vi "Test - Texture Mapping Test 1.vi"() -> ()   [LabVIEW 2020, in "3D (FPGA).lvlib"]
uses:
  3D (FPGA).lvlib
  Libraries/Utility/Utility.lvlib
  Raster/Raster (FPGA).lvlib
  Vector 3D.ctl
  Triangle 3D With Colour.ctl
  Raster/Rectangle Dimensions.ctl
  Camera.ctl
panel:
  in  "x Rotation":sgl(slide) scale=-180.0..180.0
  in  "y Rotation":sgl(slide) scale=0.0..360.0
  in  "z Rotation":sgl(slide) scale=-180.0..180.0
  in  "x Transform":sgl(slide) scale=-10.0..10.0
  in  "y Transform":sgl(slide)=5.0 scale=-10.0..10.0
  in  "z Transform":sgl(slide)=-10.0 scale=-20.0..10.0
  out "2D Picture 2":picture
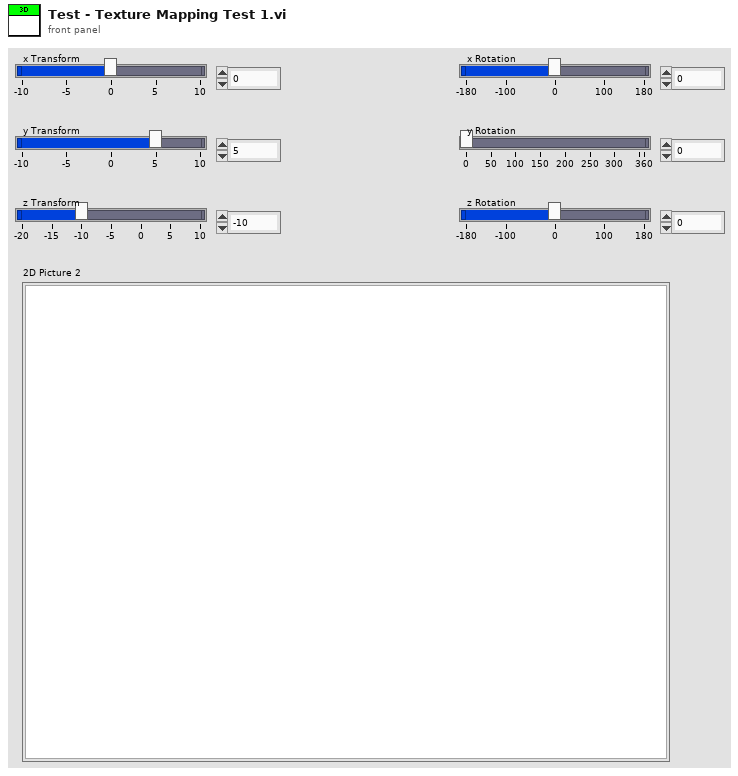
[diagram p1: front panel]
types:
  T1 = typedef "3D (FPGA).lvlib/Vector 3D.ctl" = cluster{"x":sgl, "y":sgl, "z":sgl}
  T2 = typedef "3D (FPGA).lvlib/Camera.ctl" = cluster{"Field Of View":sgl, "Near Plane":sgl, "Far Plane":sgl}
  T3 = typedef "Raster (FPGA).lvlib/Rectangle Dimensions.ctl" = cluster{"Width":u32, "Height":u32}
  T4 = typedef "3D (FPGA).lvlib/Object.ctl" = cluster{"Triangles":T5[], "Transform":T10, "Name":string, "Alpha Blending Enabled":bool, "Alpha":dbl, "Turntable Enabled":bool, "Material":T8}
  T5 = typedef "3D (FPGA).lvlib/Triangle.ctl" = cluster{"Vertex 1":T6, "Vertex 2":T6, "Vertex 3":T6, "Alpha":dbl, "Alpha Blending Enabled":bool, "Colour":u32, "Material":T8}
  T6 = typedef "3D (FPGA).lvlib/Vertex.ctl" = cluster{"Position":T1, "UV":T7, "Colour":u32}
  T7 = typedef "Raster (FPGA).lvlib/UV.ctl" = cluster{"u":sgl, "v":sgl}
  T8 = typedef "3D (FPGA).lvlib/Material.ctl" = cluster{"Diffuse Colour":u32, "Texture":T9}
  T9 = typedef "Raster (FPGA).lvlib/Texture.ctl" = cluster{"Pixels":refnum<data-value>, "Size":T3}
  T10 = typedef "3D (FPGA).lvlib/Transform.ctl" = cluster{"Position":T1, "Rotation":T1, "Scale":T1}
  T11 = typedef "3D.lvlib/Triangle 3D.ctl" = cluster{"Point 1":T12, "Point 2":T12, "Point 3":T12}
  T12 = typedef "3D.lvlib/Vector 3D.ctl" = cluster{"x":sgl, "y":sgl, "z":sgl}
  T13 = typedef "imagedata.ctl" = cluster{"image type":i32, "image depth":i32, "image":u8[], "mask":u8[], "colors":u32[], "Rectangle":cluster{"left":i16, "top":i16, "right":i16, "bottom":i16}}
  T14 = typedef "3D (FPGA).lvlib/Triangle 3D With Colour.ctl" = cluster{"Point 1":T1, "Point 2":T1, "Point 3":T1, "Fill Colour":u32, "Alpha":dbl, "Alpha Blending Enabled":bool, "Index":i32}
  T15 = typedef "3D.lvlib/Point 2D.ctl" = cluster{"x":sgl, "y":sgl}
  T16 = typedef "Raster.lvlib/UV.ctl" = cluster{"u":sgl, "v":sgl}
  T17 = typedef "Raster (FPGA).lvlib/Point 2D (I32).ctl" = cluster{"x":i32, "y":i32}
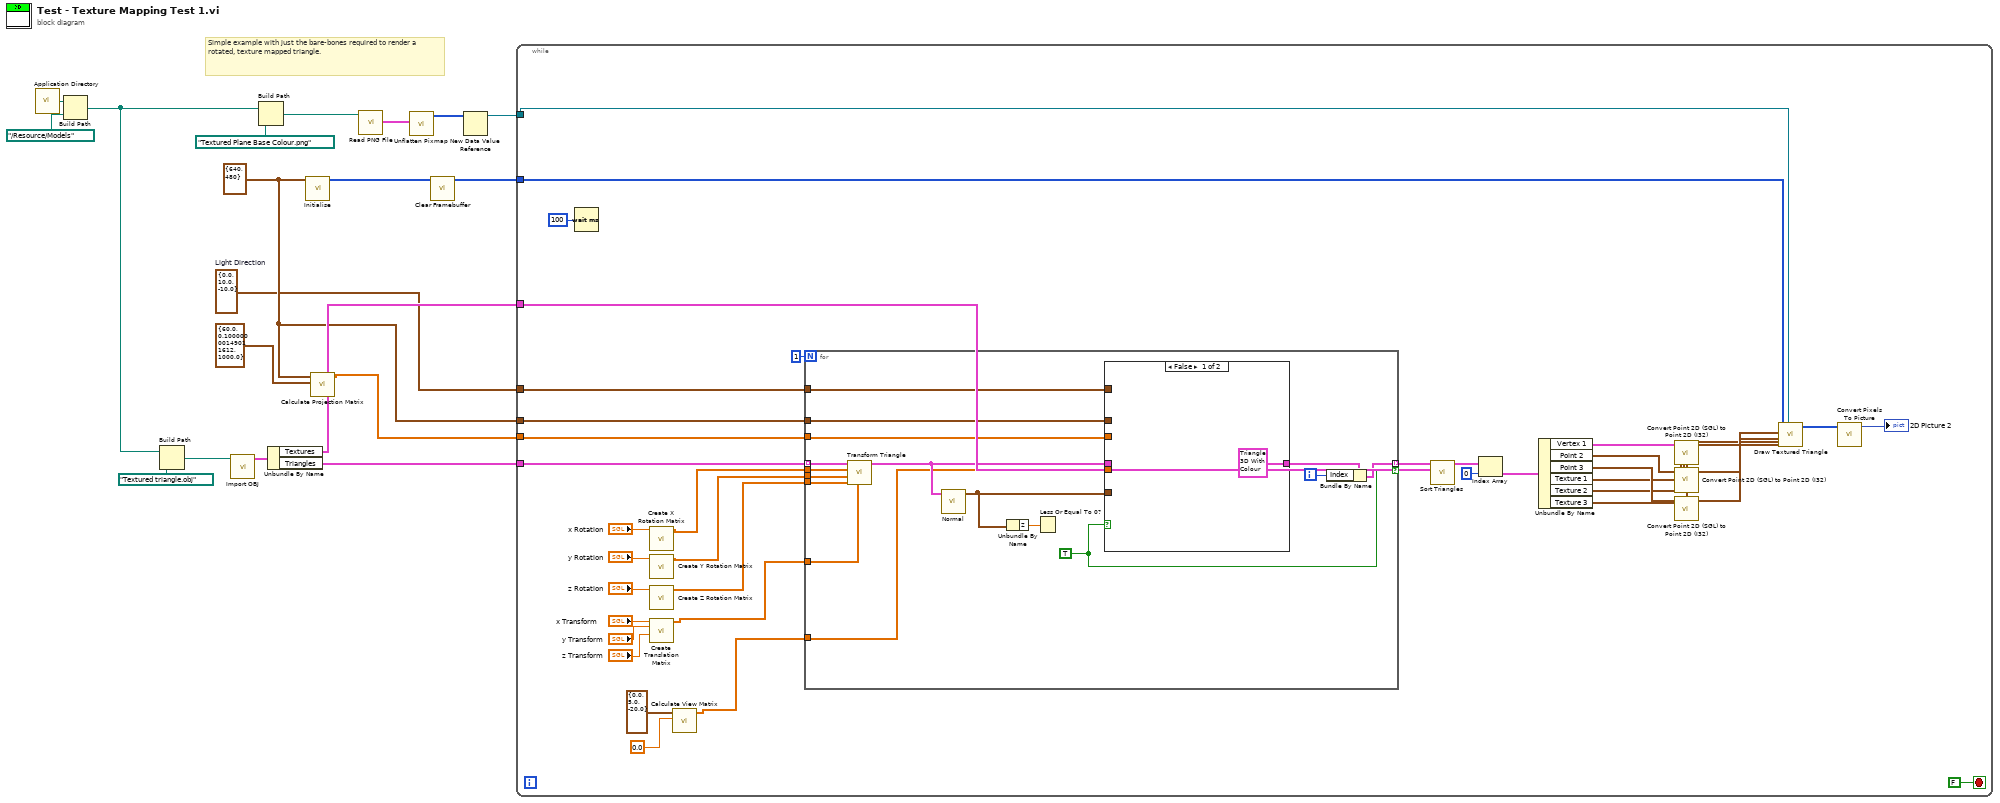
[diagram p0: block diagram]
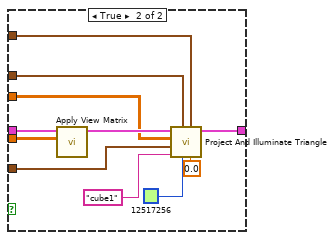
[diagram p2: hidden frame]
diagram:
  w13 = T1 {"x"=0.0, "y"=10.0, "z"=-10.0}  # Light Direction
  w14 = T3 {"Width"=640, "Height"=480} ("Screen Dimensions")
  # "Simple example with just the bare-bones required to render a rotated, texture mapped triangle."
  n1 = call <vilib>:"Application Directory.vi"() -> ("Application Directory"=w11:path)
  n2 = Build Path(base path=w11, name or relative path=path "../Resource/Models") -> (appended path=w5:path)
  n3 = Build Path(base path=w5, name or relative path=path "Textured triangle.obj") -> (appended path=w8:path)
  n4 = call "Import OBJ.vi"("Object"=w8) -> ("Object"=w18:T4)  [unwired: 9 in, 1 out]
  n5 = Build Path(base path=w5, name or relative path=path "Textured Plane Base Colour.png") -> (appended path=w6:path)
  n6 = Unbundle By Name(w18) -> ("Textures"=w15:T11[], "Triangles"=w1:T5[])
  n7 = call "Initialise.vi"("Screen Dimensions"=w14) -> ("Pixel Data out"=w16:u32[][])  [unwired: 10 in]
  n8 = call "Calculate Projection Matrix.vi"("Camera"=T2 {"Field Of View"=60.0, "Near Plane"=0.1, "Far Plane"=1000.0}, "Screen Dimensions"=w14) -> ("Projection Matrix"=w12:sgl[][])  [unwired: 9 in]
  n9 = call <vilib>:"Read PNG File.vi"("path to PNG file"=w6) -> ("image data"=w3:T13)  [unwired: 8 in, 2 out]
  n10 = call <vilib>:"Unflatten Pixmap.vi"("image data"=w3) -> ("24-bit pixmap"=w4:u32[][])  [unwired: 4 in, 6 out]
  n11 = call "Clear Framebuffer.vi"("Pixel Data in"=w16) -> ("Pixel Data out"=w19:u32[][])  [unwired: 10 in]
  n12 = New Data Value Reference(data value=w4) -> (data value reference=w2:refnum<data-value>)  [unwired: 1 in, 1 out]
  n13 = while {
    tunnel: w19 -> [w56]
    tunnel: w15 -> [w31]
    tunnel: w14 -> [w29]
    tunnel: w13 -> [w28]
    tunnel: w12 -> [w27]
    tunnel: w2 -> [w23]
    tunnel: w1 -> [w22]
    stop <- FALSE stop-if-true
    n14 = Wait (ms)(milliseconds to wait=u32 100) -> ()  [unwired: 1 out]
    n15 = call "Create X Rotation Matrix.vi"("Theta (°)"="x Rotation") -> ("Rotation X Matrix"=w39:sgl[][])  [unwired: 10 in]
    n16 = call "Create Y Rotation Matrix.vi"("Theta (°)"="y Rotation") -> ("Rotation Y Matrix"=w38:sgl[][])  [unwired: 10 in]
    n17 = call "Create Z Rotation Matrix.vi"("Theta (°)"="z Rotation") -> ("Rotation Z Matrix"=w37:sgl[][])  [unwired: 10 in]
    n18 = call "Create Translation Matrix.vi"("z"="z Transform", "y"="y Transform", "x"="x Transform") -> ("Translation Matrix"=w36:sgl[][])  [unwired: 8 in]
    n19 = call "Calculate View Matrix.vi"("Camera Rotation"=sgl 0.0, "Camera Position"=T1 {"x"=0.0, "y"=5.0, "z"=-20.0} ("output cluster")) -> ("View Matrix"=w33:sgl[][])  [unwired: 9 in]
    n20 = for {
      N: 1 -> [_]
      tunnel: w37 -> [w70]
      tunnel: w39 -> [w72]
      tunnel: [w60] -> w32 mode=indexing if=w58
      tunnel: w38 -> [w71]
      tunnel: w36 -> [w69]
      tunnel: w22 -> [w62] mode=indexing
      tunnel: w29 -> [w67]
      tunnel: w27 -> [w66]
      tunnel: w28 -> [w65]
      tunnel: w33 -> [w63]
      i -> [w59]
      w58 = TRUE
      n21 = call "Transform Triangle.vi"("Translation Matrix"=w69, "Rotation Z Matrix"=w70, "Rotation Y Matrix"=w71, "Rotation X Matrix"=w72, "Triangle in"=w62) -> ("Triangle out"=w68:T5)  [unwired: 6 in]
      n22 = call "Normal.vi"("Triangle"=w68) -> ("Normal"=w73:T1)  [unwired: 10 in]
      n23 = Unbundle By Name(w73) -> ("z"=w64:sgl)
      n24 = Less Or Equal To 0?(x=w64) -> ()  [unwired: 1 out]
      n25 = case shown="False" w58 {
        tunnel: [T14 {"Point 1"={"x"=0.0, "y"=0.0, "z"=0.0}, "Point 2"={"x"=0.0, "y"=0.0, "z"=0.0}, "Point 3"={"x"=0.0, "y"=0.0, "z"=0.0}, "Fill Colour"=12517256, "Alpha"=0.0, "Alpha Blending Enabled"=FALSE, "Index"=0} ("Triangle") w79] -> w61
        tunnel: w73 -> [_ w85]
        tunnel: w68 -> [_ w83]
        tunnel: w67 -> [_ w82]
        tunnel: w66 -> [_ w81]
        tunnel: w65 -> [_ w80]
        tunnel: w63 -> [_ w78]
        frame False {
        }
        frame True {
          n26 = call "Apply View Matrix.vi"("View Matrix"=w78, "Triangle in"=w83) -> ("Triangle out"=w84:T5)  [unwired: 9 in]
          n27 = call "Project And Illuminate Triangle.vi"("Alpha"=0.0, "Light Direction"=w80, "Diffuse Colour"=u32 12517256, "Screen Dimensions"=w82, "Name"="cube1", "Normal"=w85, "Projection Matrix"=w81, "Triangle in"=w84) -> ("Triangle out"=w79:T5)  [unwired: 3 in]
        }
      }
      n28 = Bundle By Name(cluster=w61, "Index"=w59) -> (w60:T5)
    }
    n29 = call "Sort Triangles.vi"(10:w31, "Triangles"=w32) -> ("Triangles Sorted"=w30:T5[])  [unwired: 9 in]
    n30 = Index Array(array=w30, index=0) -> (element=w52:T5)
    n31 = Unbundle By Name(w52) -> ("Vertex 1"=w55:T6, "Point 2"=w54:T15, "Point 3"=w53:T15, "Texture 1"=w47:T16, "Texture 2"=w46:T16, "Texture 3"=w45:T16)
    n32 = call "Convert Point 2D (SGL) to Point 2D (I32).vi"("Point 2D (Float)"=w55) -> ("Point 2D (I32)"=w50:T17)  [unwired: 10 in]
    n33 = call "Convert Point 2D (SGL) to Point 2D (I32).vi"("Point 2D (Float)"=w54) -> ("Point 2D (I32)"=w49:T17)  [unwired: 10 in]
    n34 = call "Convert Point 2D (SGL) to Point 2D (I32).vi"("Point 2D (Float)"=w53) -> ("Point 2D (I32)"=w48:T17)  [unwired: 10 in]
    n35 = call "Draw Textured Triangle.vi"(0:w45, 4:w46, 6:w47, 7:w23, 8:w48, "Texture"=w49, "Triangle"=w50, "Pixel Data in"=w56) -> ("Pixel Data out"=w24:u32[][])  [unwired: 3 in]
    n36 = call "Convert Pixels To Picture.vi"("Pixel Data in"=w24) -> ("2D Picture"=→"2D Picture 2":picture)  [unwired: 9 in, 1 out]
  }
